vi "Auto Calibration.vi"(4 "Run Optimization Proc":bool, 5 "HasESI2":bool=TRUE, 6 "HasESI1":bool=TRUE, 7 "CalOption":enum32{"Positive", "Negative"}(radio)) -> (0 "error out":errorcluster)   [LabVIEW 2015]
uses:
  Type/_CalibrationStep.ctl
  Type/_GUI Method.ctl
  Type/_Lens Property.ctl
  Type/_Mass Range Property.ctl
  Type/_Mass Range Parameters.ctl
  Type/_RT Res Type.ctl
  Type/_Run Mode.ctl
  Type/_Instrument Model.ctl
  Controls/Auto-Detector Bias Info.ctl
  Controls/Auto-Detector Peak Info.ctl
  Type/_Log Command.ctl
  Type/_Data Operation.ctl
  Type/_RT Command.ctl
  Type/_CalibrationResult.ctl
  Type/_SaveOption.ctl
  Configuration/_Global Configuration.vi
  <vilib>/Utility/config.llb/Read Key (String).vi
  <vilib>/Utility/config.llb/Write Key (String).vi
  <vilib>/Utility/config.llb/NI_LVConfig.lvlib
panel:
  out "Q1 Data":string[][](array[string])
  out "Completed":bool=TRUE
  out "DV Optimization Run":string="Peak Width At (%): 50\nSearch Range (amu): +/- 2\nThreshold (counts): 1000\n"
  out "CalOption 2":enum32{"Positive", "Negative"}(ring)
  out "PeakWidth":cluster{"RefMass":dbl[], "PeakWidth":dbl[]}(graph) caption="EMS+Q1, Mass 59.06, EV30"
  out "MassShift":cluster{"RefMass":dbl[], "MassShift":dbl[]}(graph) caption="EMS+Q1, Mass 59.06, EV30"
  out "Resolution":string[][](table)=[["Quadrupole 1", "15"], ["Quadrupole 2", "3000"]]
  out "Iteration #":i32
  in  "Print":bool
  in  "Pause":bool
  out "Current Scan #":i32
  out "Calibration State":T1=enum."Get Cal Files"
  out "ScanMode":string="For Q1 Positive Mode"
  out "Detector":string[][](table)=[["Detector Deflector", "15"], ["Discriminator", "12"], ["Detector Voltage", "2350"], ["Detector Horn", "5500"]]
  out "Source":string[][](table)=[["Drying Gas", "40"], ["Nebulizer Gas 1", "0"], ["Heating Gas 1", "0"], ["Nebulizer Gas 2", "100"], ["Heating Gas 2", "0"], ["Source Exhaust", "0"], ["HSID Temperature", "200"], ["Source 1 Temp", "0"], ["Source 2 Temp", "0"], ["ElectroSpray V1", "3850"], ["ElectroSpray V2", "3850"], ["Curtain Cap", "1000"]]
  out "Instrument":string[][](table)=[["Multipole 1 RF", "350"], ["Entrance Voltage", "35"], ["Entrance Deflector", "0"], ["Multipole 1", "5"], ["Multipole Lens 1", "0"], ["Multipole 2", "0"], ["Multipole Lens 2", "0"], ["Prefilter", "-15"], ["Collision Cell Lens 1", "-10"], ["Collision Cell Lens 2", "-100"], ["Collision Energy", "-50"], ["Axial Field", "100"], ["Collision Cell Lens 3", "-120"], ["Collision Cell Lens 4", "-65"], ["Collision Pressure", "0"]]
  out "SearchParam":string="Peak Width At (%): 50\nSearch Range (amu): +/- 2\nThreshold (counts): 1000\n"
  out "SystemInfo":string="Instrument Model: IONICS 3Q 220\nInstrument Serial Number: A2103536\nManufacturer: PerkinElmer\nScan Mode: Q1, Positive\nResolution: Unit_Unit\nSource: ESI2\nMethod: +Q1 PPG"
  out "DateLabel":string="Date Performed: 10/08/2013 09:12:58\nLast Performed: 09/12/2013 14:12:55"
  out "Pages":enum32{"Page 1", "Page 2", "Page 3", "Page 4"}(tab)
  out "MR 8":cluster{dbl[], dbl[]}(graph)
  out "MR 7":cluster{dbl[], dbl[]}(graph) caption="Q2 Pos, Mass 1545.13, EV70"
  out "MR 6":cluster{dbl[], dbl[]}(graph) caption="Q2 Pos, Mass 906.67, EV55"
  out "MR 5":cluster{dbl[], dbl[]}(graph) caption="Q2 Pos, Mass 616.46, EV55"
  out "MR 4":cluster{dbl[], dbl[]}(graph) caption="Q2 Pos, Mass 384.30, EV0"
  out "MR 3":cluster{dbl[], dbl[]}(graph) caption="Q2 Pos, Mass 175.13, EV55"
  out "MR 2":cluster{dbl[], dbl[]}(graph) caption="Q2 Pos, Mass 117.09, EV55"
  out "Current Results":string[][](table) caption="02/16/2017 10:53:40"
  out "MR 1":cluster{dbl[], dbl[]}(graph) caption="Q2 Pos, Mass 59.05, EV55"
  out "Previous Auto Calibration Results":string[][](table) caption="02/13/2017 14:08:53"
  out "ParmeterFolder":path
  out "ResolutionFile":path
  out "ReportFolder":path
  out "Q2ReportPage":path
  out "Q1ReportPage":path
  out "Init":bool
  out "Model Name":T2=enum."IONICS 3Q 210"
  out "UsingESI1":bool=TRUE
  out "Quit":bool
  out "oldTablePath":path
  out "Q1 Method":path=path "C:/Users/Min/Projects/SVN/Sniffer900/Release/Ionics Service Tool/Q1PositiveMethod.d2m"
  out "Q2 Method":path=path "C:/Users/Min/Projects/SVN/Sniffer900/Release/Ionics Service Tool/Q1NegativeMethod.d2m"
  in  "Page":bool=TRUE
  in  "GotoPg2":bool
  in  "GotoPg1":bool
  out "PeakSearchParameters":dbl[](array[numeric])
  out "MassReference":cluster{"Mass":dbl, "Use":bool}[](array[cluster])
  out "Method":T3={"Lenses"=[], "Mass Ranges"=[], "Acquire"=FALSE, "MCA"=FALSE, "Q1DC EN"=FALSE, "Q1 POL"=FALSE, "Q3 POL"=FALSE, "Q1 RF  EN"=FALSE, "Averaging"=FALSE, "Log Scale"=FALSE, "CPS"=FALSE, "Unit"=FALSE, "Data Path"=path "", "Run Mode"=enum."MRM (Q1/Q2)", "Fixed Mass (amu)"=1.0, "Q3DC EN"=FALSE, "Q3 RF  EN"=FALSE, "Negative"=FALSE} {"Mass Ranges"."Res" items=["High/High", "Medium/Medium", "Low/Low", "High/Medium", "High/Low", "Medium/High", "Medium/Low", "Low/High", "Low/Medium"]}
  # "Auto CAL/RES Results Report"
  # "System Information"
  # "Search Parameters"
  # "Number of Scans (Sum): 10"
  # "Page 3"
  # "Page 4"
  # "MinimumMassPeakWidth"
  # "ThresholdForMassSpectrum"
  # "SearchRange"
  # "NumberOfSmooth"
  # "NumberOfPointsToSmooth"
  # "WidthAtOfMaximum"
  # "PeakFindingNoiseLevel"
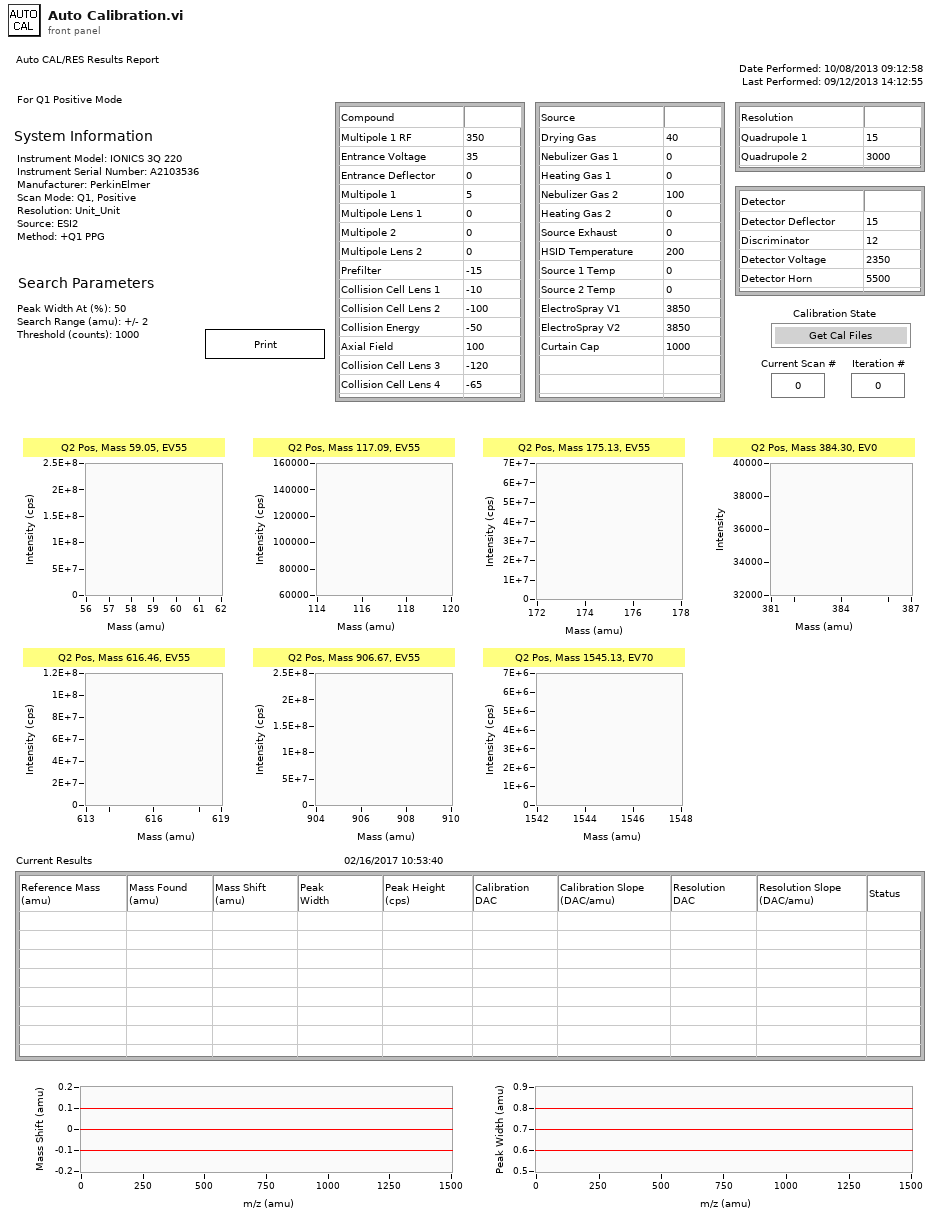
[diagram p1: front panel]
types:
  T1 = typedef "_CalibrationStep.ctl" = enum16{"Export Optimization", "Get Cal Files", "Read Q1 Method", "Acquire Q1 Data", "Process Q1 Data", "Generate Report", "Prepare For Q2 Cal", "Read Q2 Method", "Acquire Q2 Data", "Process Q2 Data", "Done", "Pause"}
  T2 = typedef "_Instrument Model.ctl" = enum16{"QSight 110", "QSight 120", "QSight 210", "QSight 220", "IONICS 3Q 110", "IONICS 3Q 120", "IONICS 3Q 210", "IONICS 3Q 220", "IONICS 3Q 310", "IONICS 3Q 320", "Simulation (Single Source)", "Simulation (Dual Source)"}
  T3 = typedef "_GUI Method.ctl" = cluster{"Lenses":T4[], "Mass Ranges":T5[], "Acquire":bool, "MCA":bool, "Q1DC EN":bool, "Q1 POL":bool, "Q3 POL":bool, "Q1 RF  EN":bool, "Averaging":bool, "Log Scale":bool, "CPS":bool, "Unit":bool, "Data Path":path, "Run Mode":T8, "Fixed Mass (amu)":dbl, "Q3DC EN":bool, "Q3 RF  EN":bool, "Negative":bool}
  T4 = typedef "_Lens Property.ctl" = cluster{"Scan Type":u8, "Scans":i32, "Time 1":dbl, "Time 2":dbl, "Value 1":dbl, "Value 2":dbl, "Step Size":dbl}
  T5 = typedef "_Mass Range Property.ctl" = cluster{"Start":dbl, "Stop":dbl, "Step Size":dbl, "Steps":i32, "Dwell":dbl, "Parameters":T6[], "Res":T7}
  T6 = typedef "_Mass Range Parameters.ctl" = cluster{"Name":string, "Ch#":u8, "StartV":dbl, "StopV":dbl, "StepV":dbl, "Index":u8}
  T7 = typedef "_RT Res Type.ctl" = u16
  T8 = typedef "_Run Mode.ctl" = enum16{"MRM (Q1/Q2)", "Q1 Scan", "Q1 SRM", "Q2 Scan", "Q2 SRM", "Product Scan", "Precursor Scan", "Neutral Loss", "Neutral Gain"}
  T9 = typedef "Auto-Detector Peak Info.ctl" = cluster{"Run Bias":u32, "Peak Height":dbl, "% Increase":dbl, "Peak Found":bool}
  T10 = typedef "Auto-Detector Bias Info.ctl" = cluster{"Run Optimization Proc":bool, "Optimization Run Bias":u32, "Run Bias Info":T9[]}
  T11 = typedef "_CalibrationResult.ctl" = cluster{"RefMass":dbl, "MassFound":dbl, "MassShift":dbl, "PeakWidth":dbl, "CalDAC":dbl, "CalSlope":dbl, "ResDAC":dbl, "ResSlope":dbl, "Status":enum16{"Found", "Missing", "Not Used"}, "CalOK":bool, "ResOK":bool, "PeakHeight":dbl}
  T12 = typedef "_Log Command.ctl" = enum16{"No Command", "Open", "Read", "Write", "Close", "Check Size"}
  T13 = typedef "_RT Command.ctl" = enum16{"xml Start Run", "xml Start Actual Run", "xml Stop Run", "xml Runtime Update", "xml Get Status", "xml Get Table", "xml Set Table", "xml Get Configuration", "xml System Status", "xml Set LC Input Logic", "xml Get Data", "xml Get Info", "Start", "StartActualRun", "Stop", "Runtime Update", "Get Data", "Get Info", "Get Status", "Get Param", "Get Config", "Get Table", "Read ADC", "Set Oscillator", "Update Config", "Update Table", "Set All Pol", "Set Pol and DC", "Set Max Mass", "Toggle RP", "Toggle EL", "Set PIC", "Initialize Turbo", "Send Turbo Comm", "Close Turbo", "P1", "P2", "P3", "Send Serial", "Set LC Out", "Get LC In", "Read VAC", "Test Table", "Toggle Power", "Get Startup", "Set Startup", "Get ADC Table", "Set ADC Table", "Get Brief Status", "Get Detail Status", "Auxiliary Update", "Set CC Logics", "Set CC Input Logics", "Ignore Error", "invalid"}
  T14 = typedef "_SaveOption.ctl" = enum16{"Use Dialog", "Temporary File", "My Tables", "Full Path"}
  T15 = typedef "_Data Operation.ctl" = enum8{"Initialize", "Get Data", "Set Data", "Close"}
  T16 = typedef "NI_LVConfig.lvlib/Config Data RefNum.ctl" = refnum<k1>
  T17 = typedef "imagedata.ctl" = cluster{"image type":i32, "image depth":i32, "image":u8[], "mask":u8[], "colors":u32[], "Rectangle":cluster{"left":i16, "top":i16, "right":i16, "bottom":i16}}
  T18 = enum16{"Left Button", "Center Button", "Right Button", "Window Close"}
  T19 = typedef "_Current Data.ctl" = cluster{"Scan#":i32, "Run Time (mS)":i32, "TIC X":dbl[], "TIC Y":dbl[][], "MassRange":cluster{"X Title":string, "X":dbl[], "Y":i32[]}[], "Fixed Mass (amu)":dbl, "Method":T20}
  T20 = typedef "_XML Expt.ctl" = cluster{"StartT(mS)":i32, "#Cycles":i32, "PauseT(uS)":i32, "ScanType":i32, "Polarity":u8, "FixedMass":dbl, "DelayT(mS)":i32, "Active Ch":T21[], "Mass Range":T5[]}
  T21 = typedef "_XML Lens.ctl" = cluster{"Value":dbl, "ChID":u8}
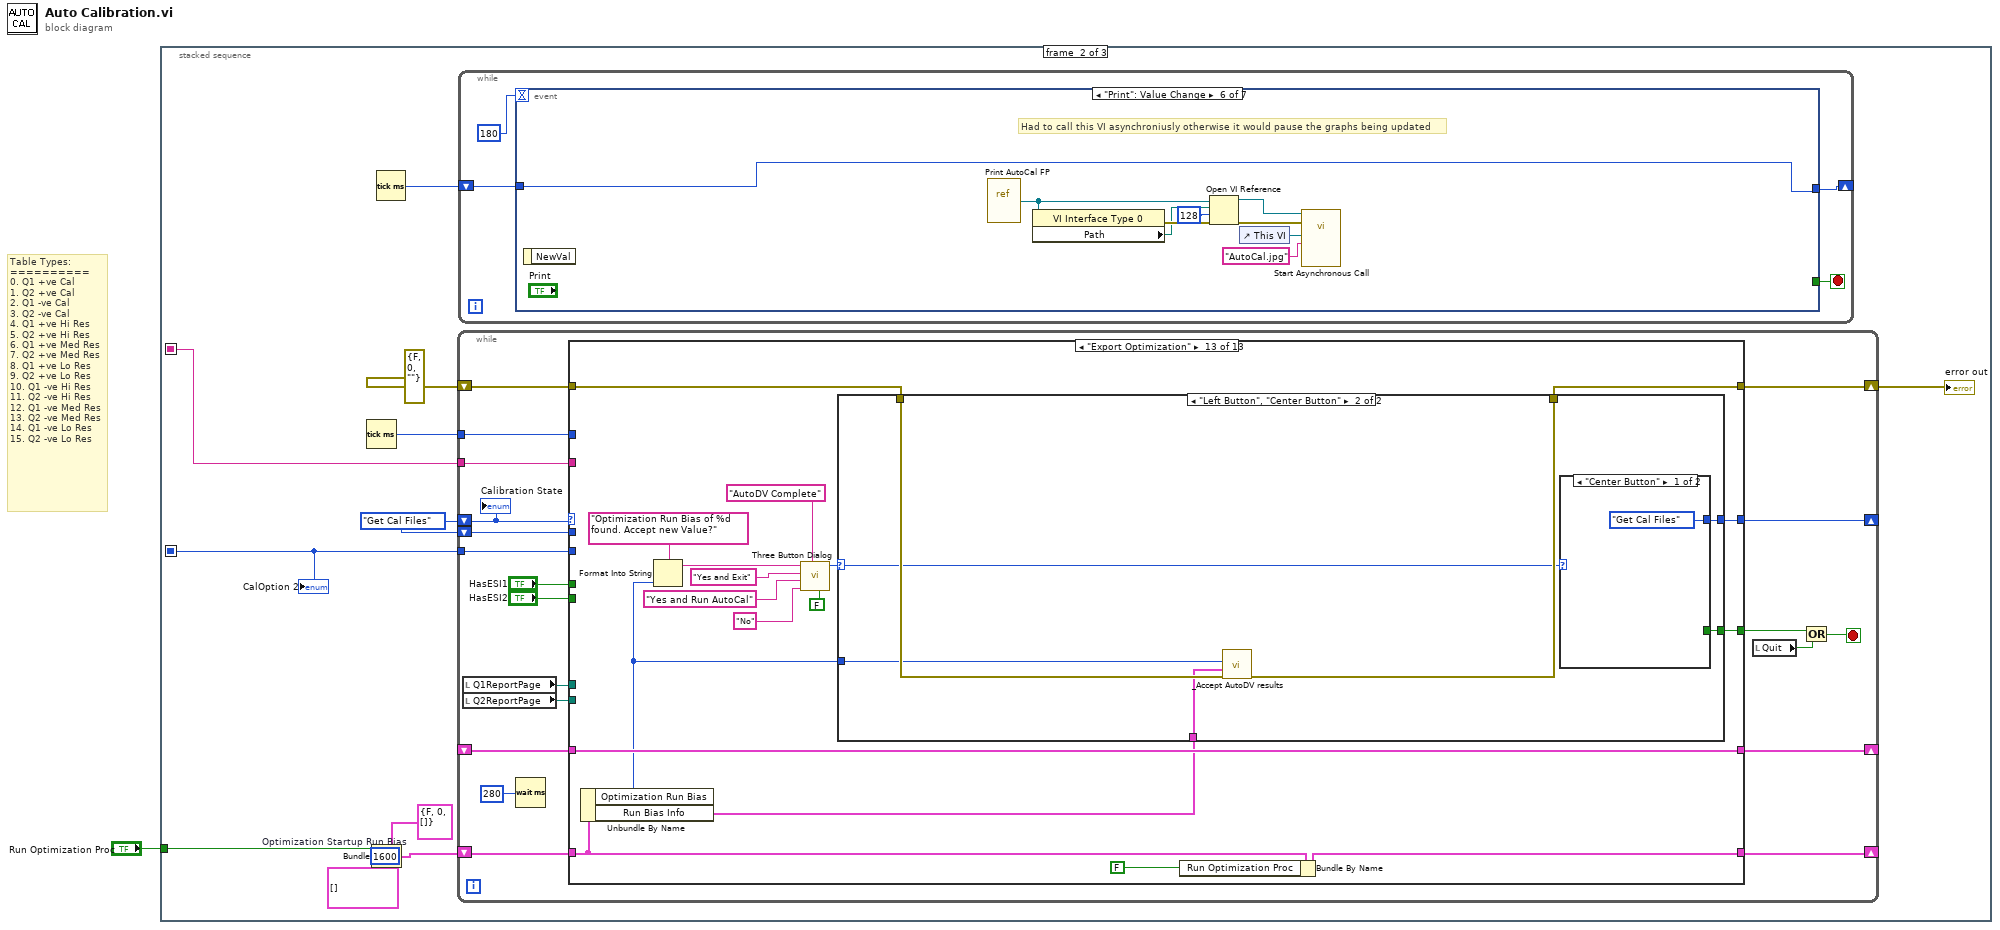
[diagram p0: block diagram]
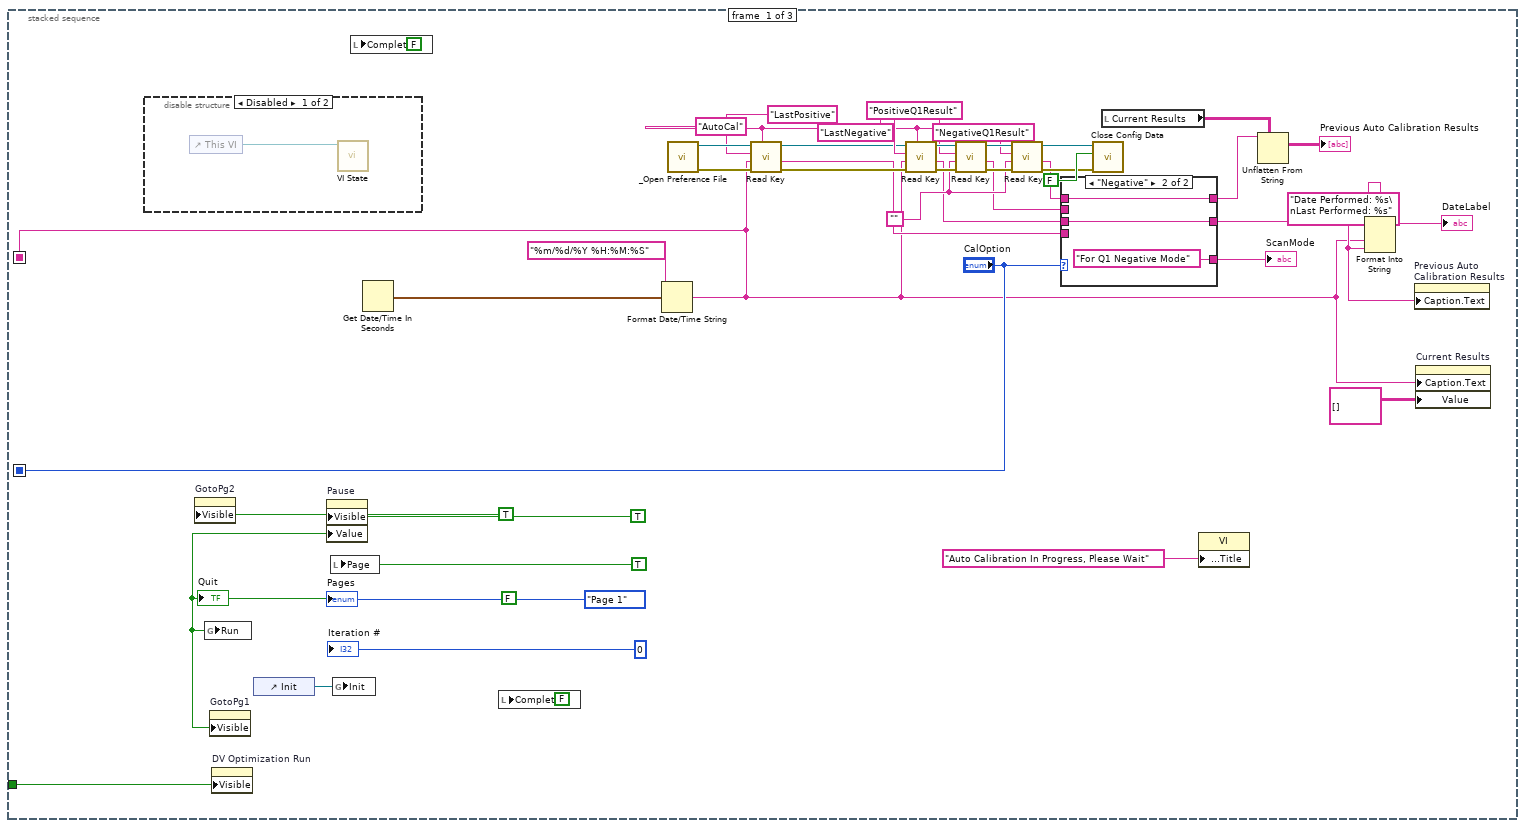
[diagram p2: hidden frame]
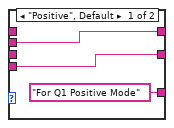
[diagram p4: hidden frame]
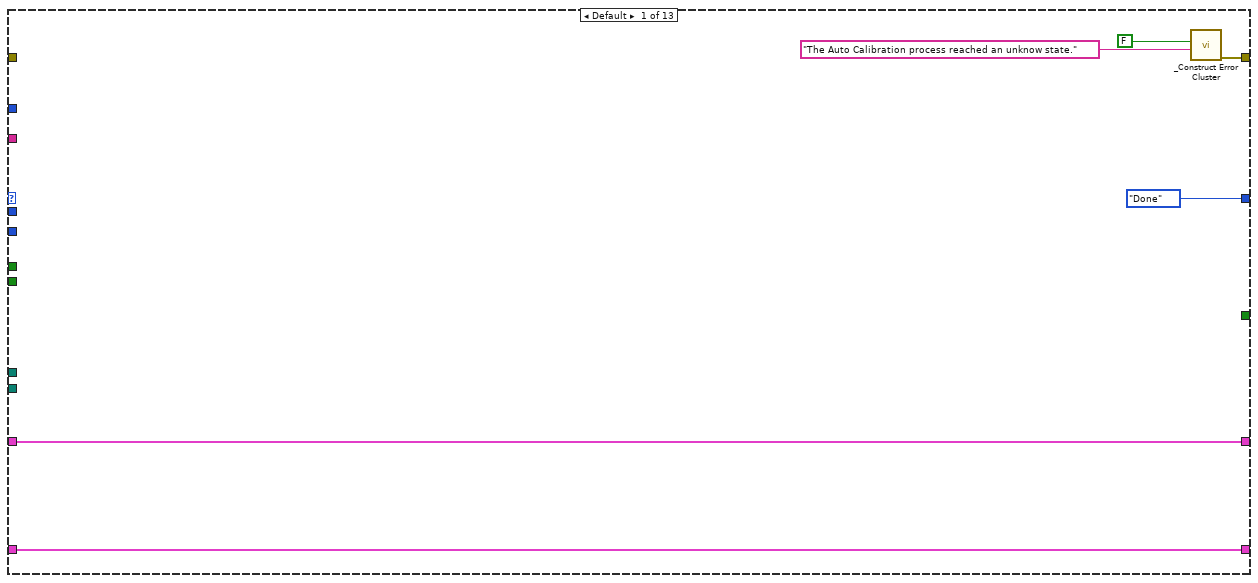
[diagram p5: hidden frame]
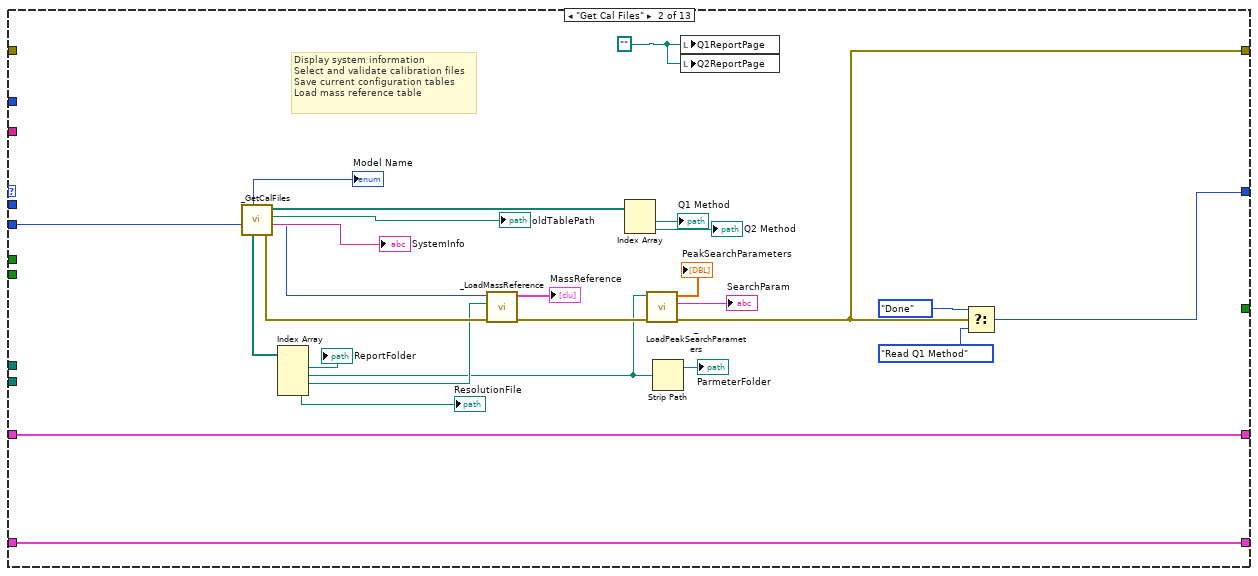
[diagram p6: hidden frame]
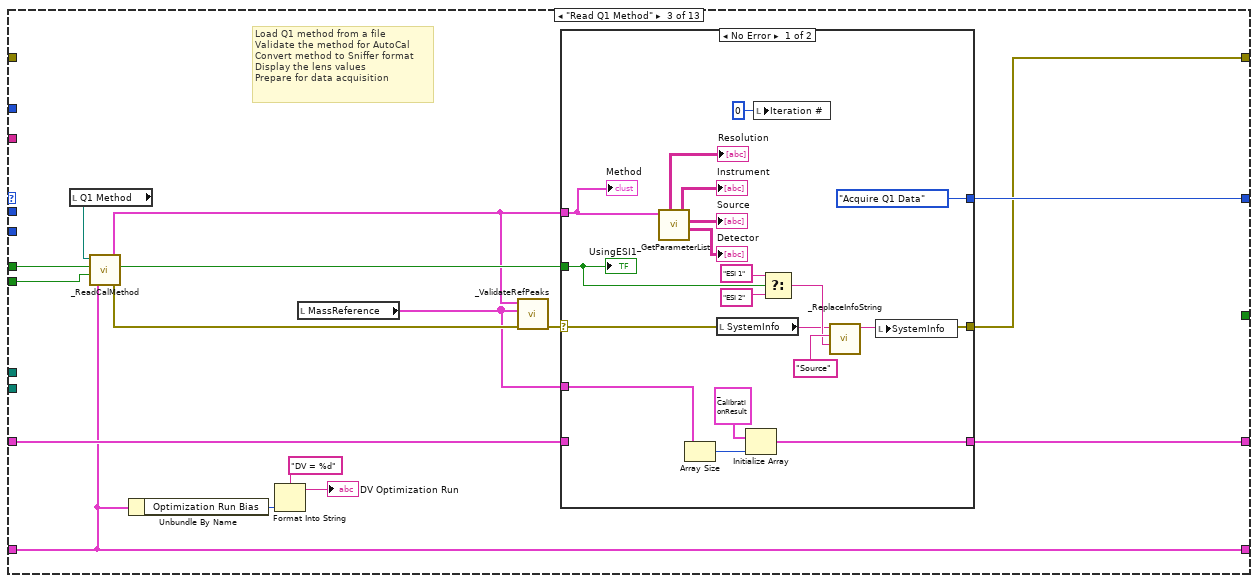
[diagram p7: hidden frame]
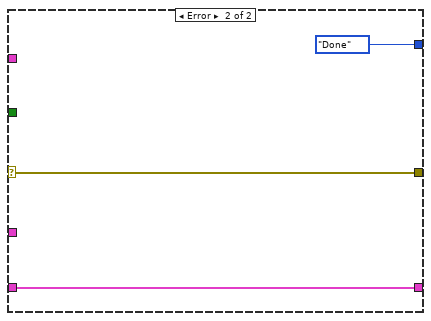
[diagram p8: hidden frame]
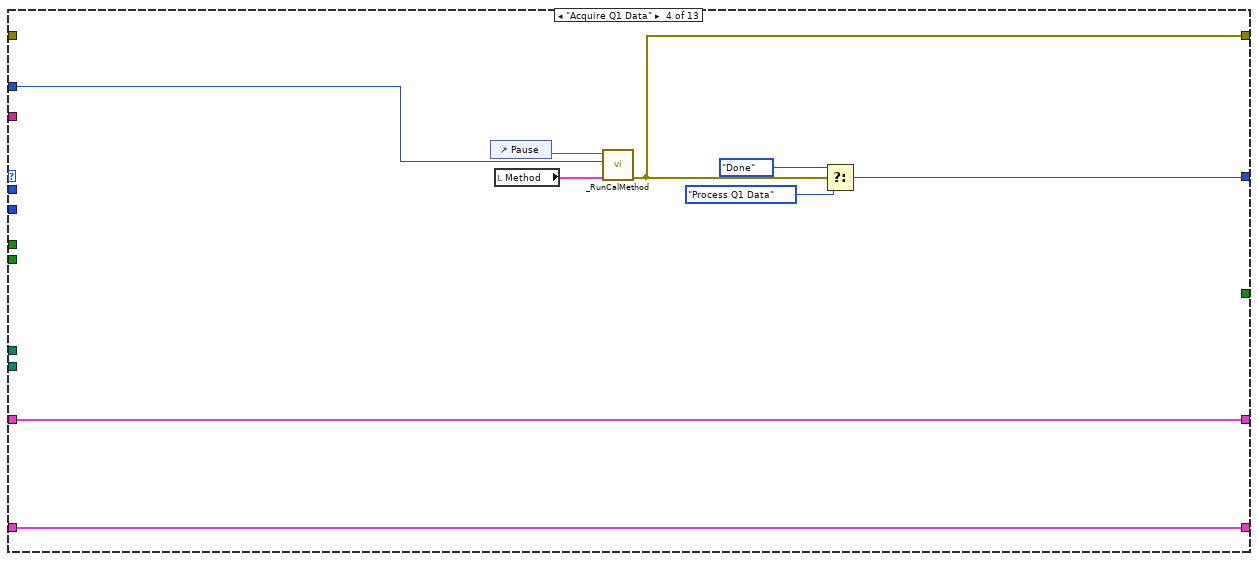
[diagram p9: hidden frame]
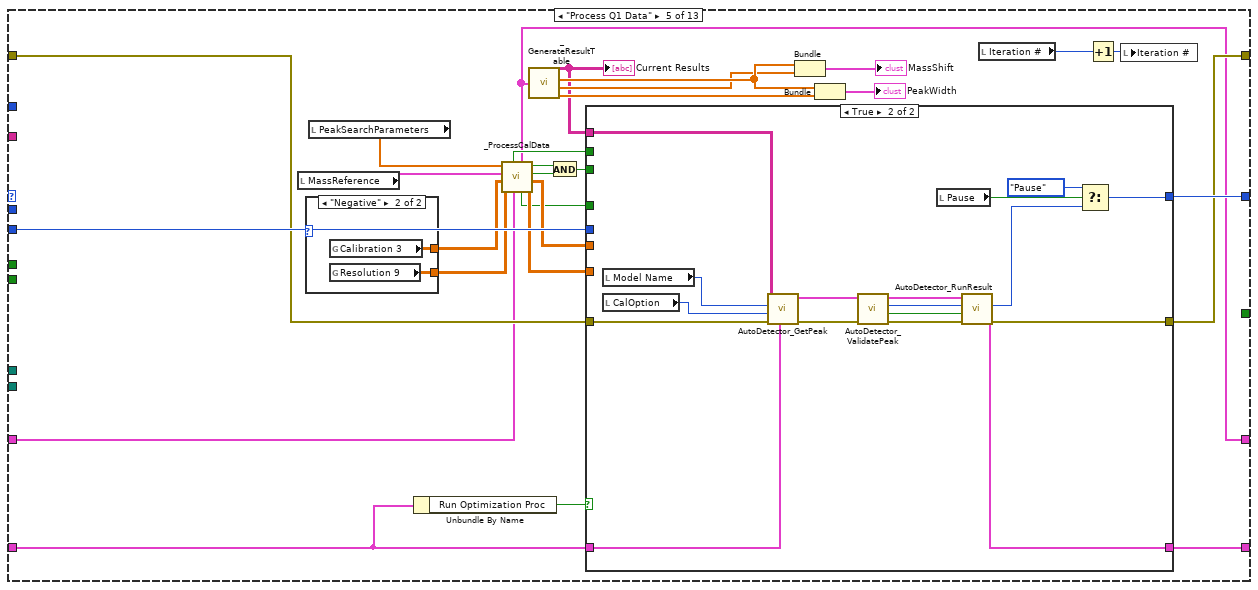
[diagram p10: hidden frame]
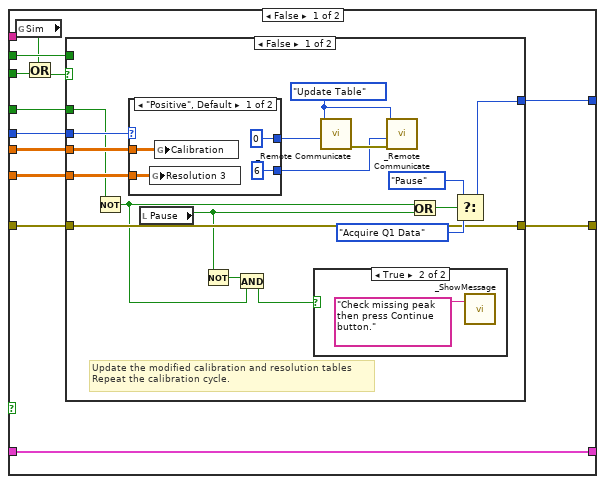
[diagram p11: hidden frame]
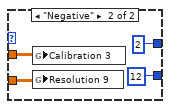
[diagram p13: hidden frame]
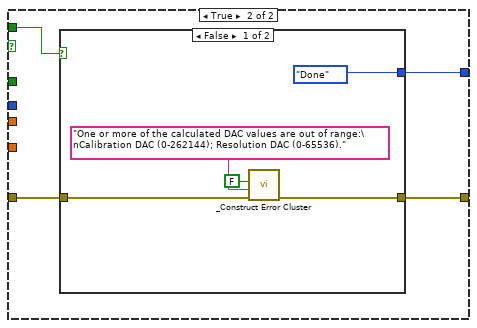
[diagram p14: hidden frame]
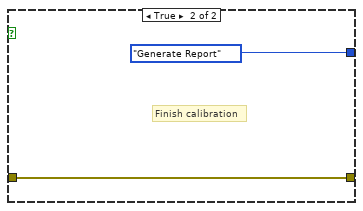
[diagram p15: hidden frame]
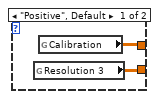
[diagram p16: hidden frame]
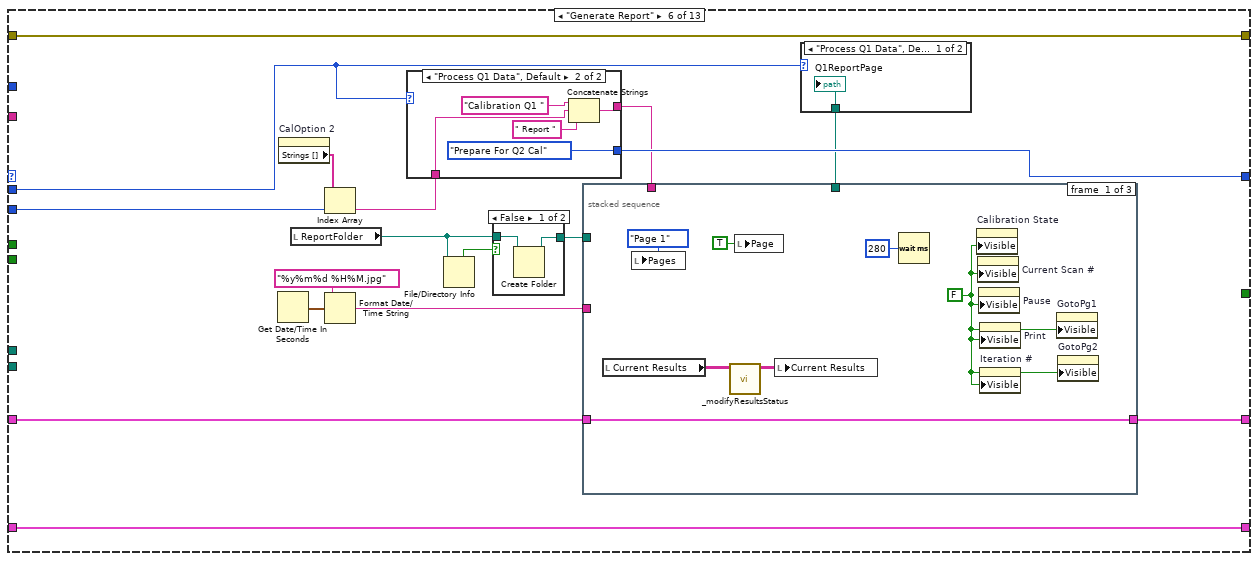
[diagram p17: hidden frame]
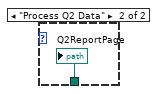
[diagram p18: hidden frame]
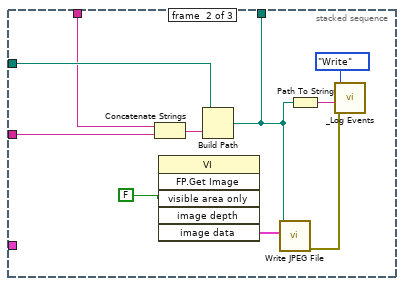
[diagram p20: hidden frame]
diagram:
  # "Table Types:\n==========\n0. Q1 +ve Cal\n1. Q2 +ve Cal\n2. Q1 -ve Cal\n3. Q2 -ve Cal\n4. Q1 +ve Hi Res\n5. Q2 +ve Hi Res\n6. Q1 +ve Med Res\n7. Q2 +ve Med Res\n8. Q1 +ve Lo Res\n9. Q2 +ve Lo Res\n10. Q1 -ve Hi Res\n11. Q2 -ve Hi Res\n12. Q1 -ve Med Res\n13. Q2 -ve Med Res\n14. Q1 -ve Lo Res\n15. Q2 -ve Lo Res"
  n1 = stacked-sequence {
    seq-local: ["CalOption" _ _] -> [_ w64 w667]
    seq-local: [w13 _ _] -> [_ w61 _]
    tunnel: "Run Optimization Proc" -> [w4 w54 _]
    frame #0 {
      w26 = ""
      w30 = "AutoCal" ("section")
      w6 = FALSE ("Quit")
      n2 = disable-structure shown="Disabled" {
        frame Disabled {
          n3 = control-ref of="This VI"() -> (w46:refnum<vi>)
          n4 = call "VI State.vi"("VI in"=w46) -> ()  [unwired: 10 in, 1 out]
        }
        frame Enabled {
        }
      }
      n5 = property on="GotoPg2" class="Bool"("Visible"=TRUE) -> ()  [unwired: 2 in, 2 out]
      n6 = global write "_Global Configuration.vi" "Run"(w6) -> ()
      n7 = property on="GotoPg1" class="Bool"("Visible"=w6) -> ()  [unwired: 2 in, 2 out]
      n8 = property on="DV Optimization Run" class="Str"("Visible"=w4) -> ()  [unwired: 2 in, 2 out]
      n9 = control-ref of="Init"() -> (w12:refnum<vi>)
      n10 = property on="Pause" class="Bool (strict)"("Visible"=TRUE, "Value"=w6) -> ()  [unwired: 2 in, 2 out]
      n11 = local write "Page"(TRUE ("Page")) -> ()
      n12 = global write "_Global Configuration.vi" "Init"(w12) -> ()
      n13 = local write "Completed"(FALSE ("Accepted")) -> ()
      n14 = Get Date/Time In Seconds() -> (seconds since 1Jan1904=w37:timestamp)
      n15 = local write "Completed"(FALSE ("Accepted")) -> ()
      n16 = Format Date/Time String(time format string (%c)="%m/%d/%Y %H:%M:%S", seconds (now)=w37) -> (date/time string=w13:string)  [unwired: 1 in]
      n17 = call "_Open Preference File.vi"() -> ("error"=w40:errorcluster, "refnum"=w44:T16)  [unwired: 3 in, 3 out]
      n18 = call-poly <vilib>:"Read Key.vi"("section"=w30, "error in (no error)"=w40, "default value"=w13, "key"="LastPositive" ("section"), "refnum"=w44) -> ("error out"=w39:errorcluster, "value"=w22:string, "refnum out"=w41:T16)  [unwired: 3 in, 1 out]
      n19 = call-poly <vilib>:"Read Key.vi"("section"=w30, "error in (no error)"=w39, "default value"=w13, "key"="LastNegative" ("section"), "refnum"=w41) -> ("error out"=w35:errorcluster, "value"=w23:string, "refnum out"=w34:T16)  [unwired: 3 in, 1 out]
      n20 = call-poly <vilib>:"Read Key.vi"("section"=w30, "error in (no error)"=w35, "default value"=w26, "key"="PositiveQ1Result" ("section"), "refnum"=w34) -> ("error out"=w32:errorcluster, "value"=w24:string, "refnum out"=w31:T16)  [unwired: 3 in, 1 out]
      n21 = call-poly <vilib>:"Read Key.vi"("section"=w30, "error in (no error)"=w32, "default value"=w26, "key"="NegativeQ1Result" ("section"), "refnum"=w31) -> ("error out"=w27:errorcluster, "value"=w25:string, "refnum out"=w28:T16)  [unwired: 3 in, 1 out]
      n22 = case shown="\"Negative\"" "CalOption" {
        tunnel: w25 -> [_ w51]
        tunnel: w24 -> [w48 _]
        tunnel: w23 -> [_ w50]
        tunnel: w22 -> [w47 _]
        tunnel: ["For Q1 Positive Mode" ("ScanMode") "For Q1 Negative Mode" ("ScanMode")] -> w21
        tunnel: [w48 w51] -> w19
        tunnel: [w47 w50] -> w15
        frame "Positive", Default {
        }
        frame "Negative" {
        }
      }
      "ScanMode" <- w21
      n23 = call <vilib>:"Close Config Data.vi"("error in (no error)"=w27, "write file if changed (T)"=FALSE, "refnum"=w28) -> ()  [unwired: 9 out]
      n24 = local read "Current Results"() -> (w20:string[][])
      n25 = property class="VI"("Front Panel Window:Title"="Auto Calibration In Progress, Please Wait") -> ()  [unwired: 2 in, 2 out]
      n26 = Unflatten From String(type=w20, binary string=w19) -> (value=→"Previous Auto Calibration Results":string[][])  [unwired: 3 in, 2 out]
      n27 = Format Into String(format string="Date Performed: %s\nLast Performed: %s", w13, w15) -> (resulting string=→"DateLabel":string)  [unwired: 2 in, 1 out]
      n28 = property on="Previous Auto Calibration Results" class="Tbl (strict)"("Caption.Text"=w15) -> ()  [unwired: 2 in, 2 out]
      n29 = property on="Current Results" class="Tbl (strict)"("Caption.Text"=w13, "Value"=string[][] [] ("Current Results")) -> ()  [unwired: 2 in, 2 out]
      "Quit" <- w6
      "Pages" <- enum32{"Page 1", "Page 2", "Page 3", "Page 4"}."Page 1" ("Pages")
      "Iteration #" <- 0 ("Iteration #")
    }
    frame #1 {
      w58 = u32 1600  # Optimization Startup Run Bias
      w62 = _CalibrationStep."Get Cal Files" ("f")
      n30 = Tick Count (ms)() -> (millisecond timer value=w55:u32)
      n31 = Bundle(cluster=T10 {"Run Optimization Proc"=FALSE, "Optimization Run Bias"=0, "Run Bias Info"=[]}, "Run Optimization Proc"=w54, "Optimization Run Bias"=w58, "Run Bias Info"=T9[] []) -> (w60:T10)
      n32 = Tick Count (ms)() -> (millisecond timer value=w53:u32)
      n33 = while {
        shift-right: [w84] -> _
        shift-left: w62 -> [w82]
        tunnel: w64 -> [w78]
        shift-right: [w76] -> w56
        shift-left: errorcluster {"status"=FALSE, "code"=0, "source"=""} ("error out 2") -> [w77]
        shift-left: w62 -> [w73]
        tunnel: w61 -> [w72]
        shift-right: [w71] -> _
        shift-left: _ -> [w70]
        shift-right: [w66] -> _
        shift-left: w60 -> [w67]
        tunnel: w55 -> [w65]
        stop <- w79 stop-if-true
        n34 = local read "Q1ReportPage"() -> (w69:path)
        n35 = local read "Q2ReportPage"() -> (w68:path)
        n36 = Wait (ms)(milliseconds to wait=u32 280) -> ()  [unwired: 1 out]
        n37 = case shown="\"Export Optimization\"" w82 {
          selector: w82 -> [_ _ _ _ _ _ _ _ _ _ w461 _ _]
          tunnel: [_CalibrationStep."Done" ("f") w112 w131 w160 w174 w276 _CalibrationStep."Read Q2 Method" ("f") w354 w383 w397 w461 w524 w550] -> w84
          tunnel: [_ _ _ _ _ _ _ _ _ _ w463 w523 w538] -> w81
          tunnel: w78 -> [_ w106 _ _ w188 w265 w332 _ _ w411 w465 _ _]
          tunnel: w77 -> [_ _ _ _ w171 w277 w333 _ _ w394 w462 w526 w549]
          tunnel: [w88 w103 w120 w161 w172 w277 w333 w342 w384 w395 w462 w526 w548] -> w76
          tunnel: "HasESI1" -> [_ _ w129 _ _ _ _ w352 _ _ _ _ _]
          tunnel: "HasESI2" -> [_ _ w128 _ _ _ _ w351 _ _ _ _ _]
          tunnel: w73 -> [_ _ _ _ _ w269 _ _ _ _ w460 w525 _]
          tunnel: w72 -> [_ _ _ _ _ _ _ _ _ _ w455 _ _]
          tunnel: [w86 w100 w123 w158 w168 w261 w314 w345 w381 w390 w459 w522 w555] -> w71
          tunnel: w70 -> [w86 w100 w124 w158 w167 w262 w314 w347 w381 w391 w459 w522 w555]
          tunnel: w69 -> [_ _ _ _ _ _ _ _ _ _ w457 _ _]
          tunnel: w68 -> [_ _ _ _ _ _ _ _ _ _ w458 _ _]
          tunnel: w67 -> [w85 w92 w119 w157 w163 w263 w313 w344 w380 w389 w456 w521 w554]
          tunnel: [w85 w92 w119 w157 w164 w263 w313 w344 w380 w389 w456 w521 w552] -> w66
          tunnel: w65 -> [_ _ _ w154 _ _ _ _ w377 _ _ _ _]
          frame Default {
            n38 = call "_Construct Error Cluster.vi"("reason"="The Auto Calibration process reached an unknow state.", "CallingChain? (T)"=FALSE) -> ("error out"=w88:errorcluster)  [unwired: 5 in]
          }
          frame "Get Cal Files" {
            w99 = path ""
            # "Display system information\nSelect and validate calibration files\nSave current configuration tables\nLoad mass reference table"
            n39 = call "_GetCalFiles.vi"("CalOption"=w106) -> ("error out"=w107:errorcluster, "SystemInfo"=→"SystemInfo":string, "oldTablePath"=→"oldTablePath":path, "calFiles"=w111:path[], "OtherDirectories"=w98:path[], "Model Name"=→"Model Name":T2)  [unwired: 3 in]
            n40 = Index Array(array=w98) -> (element #1=→"ReportFolder":path, element #2=w94:path, element #3=w97:path, element #4=→"ResolutionFile":path)  [unwired: 4 in]
            n41 = call "_LoadMassReference.vi"("error in (no error)"=w107, "Path"=w97, "Polarity"=w106) -> ("error out"=w104:errorcluster, "MassReference"=→"MassReference":cluster{"Mass":dbl, "Use":bool}[])  [unwired: 3 in]
            n42 = Index Array(array=w111) -> (element #1=→"Q1 Method":path, element #2=→"Q2 Method":path)  [unwired: 2 in]
            n43 = call "_LoadPeakSearchParameters.vi"("error in (no error)"=w104, "Path"=w94) -> ("error out"=w103:errorcluster, "SearchParameters"=→"SearchParam":string, "PeakSearchParameters"=→"PeakSearchParameters":dbl[])  [unwired: 3 in]
            n44 = Strip Path(path=w94) -> (stripped path=→"ParmeterFolder":path)  [unwired: 1 out]
            n45 = local write "Q1ReportPage"(w99) -> ()
            n46 = local write "Q2ReportPage"(w99) -> ()
            n47 = Select(t=_CalibrationStep."Done" ("f"), s=w103, f=_CalibrationStep."Read Q1 Method") -> (s? t:f=w112:T1)
          }
          frame "Read Q1 Method" {
            # "Load Q1 method from a file\nValidate the method for AutoCal\nConvert method to Sniffer format\nDisplay the lens values\nPrepare for data acquisition"
            n48 = local read "Q1 Method"() -> (w121:path)
            n49 = call "_ReadCalMethod.vi"("Auto-Detect Bias info"=w119, "HasESI2"=w128, "HasESI1"=w129, "Method Path"=w121) -> ("error out"=w127:errorcluster, "UseESI1"=w130:bool, "GUI Method"=w126:T3)  [unwired: 1 in]
            n50 = Unbundle By Name(w119) -> ("Optimization Run Bias"=w117:u32)
            n51 = Format Into String(format string="DV = %d", w117) -> (resulting string=→"DV Optimization Run":string)  [unwired: 2 in, 1 out]
            n52 = local read "MassReference"() -> (w122:cluster{"Mass":dbl, "Use":bool}[])
            n53 = call "_ValidateRefPeaks.vi"("error in (no error)"=w127, "MassReference"=w122, "Method"=w126) -> ("error out"=w125:errorcluster)  [unwired: 4 in]
            n54 = case shown="No Error" w125 {
              selector: w125 -> [w132 w151]
              tunnel: [_CalibrationStep."Acquire Q1 Data" ("f") _CalibrationStep."Done" ("f")] -> w131
              tunnel: w126 -> [w149 _]
              tunnel: w130 -> [w144 _]
              tunnel: w124 -> [_ w152]
              tunnel: [w133 w152] -> w123
              tunnel: w122 -> [w136 _]
              tunnel: [w132 w151] -> w120
              frame No Error {
                n55 = call "_GetParameterList.vi"("GUI Method"=w149) -> ("Detector"=→"Detector":string[][], "Source"=→"Source":string[][], "Instrument"=→"Instrument":string[][], "Resolution"=→"Resolution":string[][])  [unwired: 3 in, 1 out]
                n56 = Array Size(array=w136) -> (size(s)=w135:i32)
                n57 = local read "SystemInfo"() -> (w139:string)
                n58 = Initialize Array(T11 {"RefMass"=0.0, "MassFound"=0.0, "MassShift"=0.0, "PeakWidth"=0.0, "CalDAC"=0.0, "CalSlope"=0.0, "ResDAC"=0.0, "ResSlope"=0.0, "Status"=enum."Found", "CalOK"=FALSE, "ResOK"=FALSE, "PeakHeight"=0.0} ("CalResult"), w135) -> (w133:T11[])
                n59 = local write "Iteration #"(0 ("Iteration #")) -> ()
                n60 = Select(t="ESI 1", s=w144, f="ESI 2") -> (s? t:f=w140:string)
                n61 = call "_ReplaceInfoString.vi"("Value"=w140, "Key"="Source", "SystemInfo"=w139) -> ("SystemInfoOut"=w145:string)  [unwired: 4 in]
                n62 = local write "SystemInfo"(w145) -> ()
                "Method" <- w149
                "UsingESI1" <- w144
              }
              frame Error {
              }
            }
          }
          frame "Acquire Q1 Data" {
            n63 = control-ref of="Pause"() -> (w159:refnum<vi>)
            n64 = local read "Method"() -> (w162:T3)
            n65 = call "_RunCalMethod.vi"("Method"=w162, "millisecond timer value"=w154, "Pause"=w159) -> ("error out"=w161:errorcluster)  [unwired: 4 in]
            n66 = Select(t=_CalibrationStep."Done", s=w161, f=_CalibrationStep."Process Q1 Data") -> (s? t:f=w160:T1)
          }
          frame "Process Q1 Data" {
            n67 = local read "MassReference"() -> (w189:cluster{"Mass":dbl, "Use":bool}[])
            n68 = case shown="\"Negative\"" w188 {
              tunnel: [w258 w260] -> w187
              tunnel: [w257 w259] -> w186
              frame "Positive", Default {
                n69 = global read "_Global Configuration.vi" "Resolution 3"() -> (w257:dbl[][])
                n70 = global read "_Global Configuration.vi" "Calibration"() -> (w258:dbl[][])
              }
              frame "Negative" {
                n71 = global read "_Global Configuration.vi" "Calibration 3"() -> (w260:dbl[][])
                n72 = global read "_Global Configuration.vi" "Resolution 9"() -> (w259:dbl[][])
              }
            }
            n73 = local read "PeakSearchParameters"() -> (w190:dbl[])
            n74 = Unbundle By Name(w163) -> ("Run Optimization Proc"=w165:bool)
            n75 = call "_ProcessCalData.vi"("CalResultIn"=w167, "Resolution"=w186, "Calibration"=w187, "MassReference"=w189, "PeakSearchParameters"=w190) -> ("ResolutionOut"=w184:dbl[][], "CalibrationOut"=w185:dbl[][], "ResOK"=w182:bool, "CalOK"=w183:bool, "AllFound"=w175:bool, "CalResultOut"=w168:T11[], "AllValid"=w173:bool)
            n76 = call "_GenerateResultTable.vi"("CalResults"=w168) -> ("ResultTable"=w166:string[][], "RefMass"=w178:dbl[], "MassShift"=w177:dbl[], "PeakWidth"=w180:dbl[])
            "Current Results" <- w166
            n77 = And(x=w183, y=w182) -> (x .and. y?=w181:bool)
            n78 = case shown="True" w165 {
              tunnel: w188 -> [w202 _]
              tunnel: w185 -> [w201 _]
              tunnel: w184 -> [w200 _]
              tunnel: w181 -> [w199 _]
              tunnel: w175 -> [w198 _]
              tunnel: [w197 w242] -> w174
              tunnel: w173 -> [w196 _]
              tunnel: [w195 w249] -> w172
              tunnel: w171 -> [w194 w256]
              tunnel: w166 -> [_ w255]
              tunnel: [w193 w245] -> w164
              tunnel: w163 -> [w193 w246]
              frame False {
                n79 = global read "_Global Configuration.vi" "Sim"() -> (w191:bool)
                n80 = Or(x=w191, y=w199) -> (x .or. y?=w192:bool)
                n81 = case shown="False" w192 {
                  tunnel: w202 -> [w219 _]
                  tunnel: w201 -> [w218 _]
                  tunnel: w200 -> [w217 _]
                  tunnel: [w210 w232] -> w197
                  tunnel: w198 -> [w209 _]
                  tunnel: w196 -> [_ w231]
                  tunnel: [w207 w230] -> w195
                  tunnel: w194 -> [w207 w229]
                  frame False {
                    w215 = _RT_Command."Update Table" ("Command")
                    # "Update the modified calibration and resolution tables\nRepeat the calibration cycle."
                    n82 = Not(x=w209) -> (.not. x?=w204:bool)
                    n83 = case shown="\"Positive\", Default" w219 {
                      tunnel: w218 -> [w224 w228]
                      tunnel: w217 -> [w223 w227]
                      tunnel: [u16 0 ("DC Param") u16 2 ("DC Param")] -> w214
                      tunnel: [u16 6 ("DC Param") u16 12 ("DC Param")] -> w213
                      frame "Positive", Default {
                        n84 = global write "_Global Configuration.vi" "Resolution 3"(w223) -> ()
                        n85 = global write "_Global Configuration.vi" "Calibration"(w224) -> ()
                      }
                      frame "Negative" {
                        n86 = global write "_Global Configuration.vi" "Calibration 3"(w228) -> ()
                        n87 = global write "_Global Configuration.vi" "Resolution 9"(w227) -> ()
                      }
                    }
                    n88 = local read "Pause"() -> (w206:bool)
                    n89 = Not(x=w206) -> (.not. x?=w205:bool)
                    n90 = And(x=w205, y=w204) -> (x .and. y?=w203:bool)
                    n91 = case shown="True" w203 {
                      frame False {
                      }
                      frame True {
                        n92 = call "_ShowMessage.vi"("Message"="Check missing peak then press Continue button." ("message")) -> ()  [unwired: 1 in, 1 out]
                      }
                    }
                    n93 = call "_Remote Communicate.vi"("DC Param"=w214, "Command"=w215) -> ("error out"=w216:errorcluster)  [unwired: 4 in, 3 out]
                    n94 = call "_Remote Communicate.vi"("error in (no error)"=w216, "DC Param"=w213, "Command"=w215) -> ()  [unwired: 3 in, 4 out]
                    n95 = Or(x=w204, y=w206) -> (x .or. y?=w208:bool)
                    n96 = Select(t=_CalibrationStep."Pause", s=w208, f=_CalibrationStep."Acquire Q1 Data") -> (s? t:f=w210:T1)
                  }
                  frame True {
                    n97 = case shown="False" w231 {
                      tunnel: [_CalibrationStep."Done" ("t") _CalibrationStep."Generate Report" ("f")] -> w232
                      tunnel: [w234 w238] -> w230
                      tunnel: w229 -> [w233 w238]
                      frame False {
                        n98 = call "_Construct Error Cluster.vi"("error in"=w233, "reason"="One or more of the calculated DAC values are out of range:\nCalibration DAC (0-262144); Resolution DAC (0-65536).", "CallingChain? (T)"=FALSE) -> ("error out"=w234:errorcluster)  [unwired: 4 in]
                      }
                      frame True {
                        # "Finish calibration"
                      }
                    }
                  }
                }
              }
              frame True {
                n99 = local read "Model Name"() -> (w254:T2)
                n100 = local read "CalOption"() -> (w253:enum32{"Positive", "Negative"})
                n101 = call "AutoDetector_GetPeak.vi"("AutoDV Info"=w246, "error in"=w256, "CalOption"=w253, "Model Name"=w254, "Current Results"=w255) -> ("error in"=w252:errorcluster, "AutoDV Info Out"=w251:T10)  [unwired: 5 in]
                n102 = call "AutoDetector_ValidatePeak.vi"("Error In"=w252, "Auto-DV Info In"=w251) -> ("Error Out"=w250:errorcluster, "Correct Run Bias Reached"=w247:bool, "Optimized DV Value"=w244:u32, "Auto-DV Info Out"=w248:T10)  [unwired: 6 in]
                n103 = local read "Pause"() -> (w241:bool)
                n104 = call "AutoDetector_RunResult.vi"("Error In"=w250, "Correct Run Bias Reached"=w247, "Optimized DV Value"=w244, "Auto-DV Info In"=w248) -> ("Error Out"=w249:errorcluster, "Next State"=w243:T1, "Auto-DV Info Out"=w245:T10)  [unwired: 5 in]
                n105 = Select(t=_CalibrationStep."Pause", s=w241, f=w243) -> (s? t:f=w242:T1)
              }
            }
            n106 = Bundle("RefMass"=w178, "MassShift"=w177) -> (→"MassShift":cluster{"RefMass":dbl[], "MassShift":dbl[]})  [unwired: 1 in]
            n107 = Bundle("RefMass"=w178, "PeakWidth"=w180) -> (→"PeakWidth":cluster{"RefMass":dbl[], "PeakWidth":dbl[]})  [unwired: 1 in]
            n108 = local read "Iteration #"() -> (w169:i32)
            n109 = Increment(x=w169) -> (x+1=w170:i32)
            n110 = local write "Iteration #"(w170) -> ()
          }
          frame "Generate Report" {
            n111 = Get Date/Time In Seconds() -> (seconds since 1Jan1904=w273:timestamp)
            n112 = property on="CalOption 2" class="Enum (strict)"() -> ("Strings []"=w266:string[])  [unwired: 2 in, 2 out]
            n113 = local read "ReportFolder"() -> (w267:path)
            n114 = Index Array(array=w266, index=w265) -> (element=w264:string)
            n115 = Format Date/Time String(time format string (%c)="%y%m%d %H%M.jpg", seconds (now)=w273) -> (date/time string=w272:string)  [unwired: 1 in]
            n116 = case shown="\"Process Q1 Data\", Default" w269 {
              tunnel: [w303 w306] -> w275
              tunnel: [_CalibrationStep."Done" ("f") _CalibrationStep."Prepare For Q2 Cal" ("f")] -> w276
              tunnel: w264 -> [w302 w308]
              frame "Process Q2 Data" {
                n117 = Concatenate Strings("Calibration Q2 " ("time format string (%c)"), w302, " Report " ("string")) -> (w303:string)
              }
              frame "Process Q1 Data", Default {
                n118 = Concatenate Strings("Calibration Q1 " ("time format string (%c)"), w308, " Report " ("string")) -> (w306:string)
              }
            }
            n119 = File/Directory Info(path=w267) -> (directory=w271:bool)  [unwired: 1 in, 6 out]
            n120 = case shown="False" w271 {
              tunnel: w267 -> [w281 w282]
              tunnel: [w280 w282] -> w270
              frame False {
                n121 = Create Folder(path (use dialog)=w281) -> (created path=w280:path)  [unwired: 2 in, 2 out]
              }
              frame True {
              }
            }
            n122 = stacked-sequence {
              tunnel: w270 -> [_ w296 _]
              tunnel: w275 -> [_ w295 _]
              tunnel: w272 -> [_ w294 _]
              tunnel: [_ w290 _] -> w268
              tunnel: w262 -> [w285 _ _]
              tunnel: [w285 _ _] -> w261
              frame #0 {
                w286 = FALSE ("Visible")
                n123 = local read "Current Results"() -> (w284:string[][])
                n124 = local write "Pages"(enum32{"Page 1", "Page 2", "Page 3", "Page 4"}."Page 1" ("Pages")) -> ()
                n125 = call "_modifyResultsStatus.vi"("Current Results In"=w284) -> ("Current Results Out"=w283:string[][])  [unwired: 10 in]
                n126 = local write "Page"(TRUE ("Page")) -> ()
                n127 = local write "Current Results"(w283) -> ()
                n128 = Wait (ms)(milliseconds to wait=u32 280) -> ()  [unwired: 1 out]
                n129 = property on="Calibration State" class="Enum (strict)"("Visible"=w286) -> ()  [unwired: 2 in, 2 out]
                n130 = property on="Current Scan #" class="DigNum (strict)"("Visible"=w286) -> ()  [unwired: 2 in, 2 out]
                n131 = property on="Pause" class="Bool (strict)"("Visible"=w286) -> ()  [unwired: 2 in, 2 out]
                n132 = property on="Print" class="Bool"("Visible"=w286) -> ()  [unwired: 2 in, 2 out]
                n133 = property on="Iteration #" class="DigNum (strict)"("Visible"=w286) -> ()  [unwired: 2 in, 2 out]
                n134 = property on="GotoPg1" class="Bool"("Visible"=w286) -> ()  [unwired: 2 in, 2 out]
                n135 = property on="GotoPg2" class="Bool"("Visible"=w286) -> ()  [unwired: 2 in, 2 out]
              }
              frame #1 {
                n136 = Concatenate Strings(w295, w294) -> (w297:string)
                n137 = invoke class="VI" method="FP.Get Image"("visible area only"=FALSE ("Visible Area Only")) -> ("image data"=w299:T17)  [unwired: 5 in, 5 out]
                n138 = Build Path(base path=w296, name or relative path=w297) -> (appended path=w290:path)
                n139 = call <vilib>:"Write JPEG File.vi"("image data"=w299, "path to JPEG file"=w290) -> ("error out"=w291:errorcluster)  [unwired: 1 in, 8 out]
                n140 = Path To String(path=w290) -> (string=w293:string)
                n141 = call "_Log Events.vi"("error in (no error)"=w291, "Event"=w293, "Log Command"=_Log_Command."Write") -> ()  [unwired: 5 in, 2 out]
              }
              frame #2 {
                w300 = TRUE ("Visible")
                n142 = property on="Calibration State" class="Enum (strict)"("Visible"=w300) -> ()  [unwired: 2 in, 2 out]
                n143 = property on="Pause" class="Bool (strict)"("Visible"=w300) -> ()  [unwired: 2 in, 2 out]
                n144 = property on="Print" class="Bool"("Visible"=w300) -> ()  [unwired: 2 in, 2 out]
                n145 = property on="Current Scan #" class="DigNum (strict)"("Visible"=w300) -> ()  [unwired: 2 in, 2 out]
                n146 = property on="Iteration #" class="DigNum (strict)"("Visible"=w300) -> ()  [unwired: 2 in, 2 out]
              }
            }
            n147 = case shown="\"Process Q1 Data\", Default" w269 {
              tunnel: w268 -> [w278 w279]
              frame "Process Q1 Data", Default {
                "Q1ReportPage" <- w278
              }
              frame "Process Q2 Data" {
                "Q2ReportPage" <- w279
              }
            }
          }
          frame "Prepare For Q2 Cal" {
            # "Save Q1 calibration result table\nLoad the previous Q2 calibration result table"
            n148 = case shown="\"Positive\", Default" w332 {
              tunnel: ["For Q2 Positive Mode" ("ScanMode") "For Q2 Negative Mode" ("ScanMode")] -> w323
              tunnel: ["Q2, Positive" ("time format string (%c)") "Q2, Negative" ("time format string (%c)")] -> w317
              tunnel: ["Q2 PPG POS Default.method" ("time format string (%c)") "Q2 PPG NEG Default.method" ("time format string (%c)")] -> w319
              tunnel: ["PositiveQ2Result" ("section") "NegativeQ2Result" ("section")] -> w311
              frame "Positive", Default {
              }
              frame "Negative" {
              }
            }
            n149 = local read "Current Results"() -> (w312:string[][])
            "Q1 Data" <- w312
            n150 = call "_Open Preference File.vi"() -> ("error"=w330:errorcluster, "refnum"=w331:T16)  [unwired: 3 in, 3 out]
            n151 = local read "SystemInfo"() -> (w320:string)
            n152 = local write "ScanMode"(w323) -> ()
            n153 = call "_ReplaceInfoString.vi"("Value"=w319, "Key"="Method", "SystemInfo"=w320) -> ("SystemInfoOut"=w318:string)  [unwired: 4 in]
            n154 = call-poly <vilib>:"Read Key.vi"("section"="AutoCal", "error in (no error)"=w330, "default value"="", "key"=w311, "refnum"=w331) -> ("error out"=w328:errorcluster, "value"=w325:string, "refnum out"=w329:T16)  [unwired: 3 in, 1 out]
            n155 = call "_ReplaceInfoString.vi"("Value"=w317, "Key"="Scan Mode", "SystemInfo"=w318) -> ("SystemInfoOut"=w315:string)  [unwired: 4 in]
            n156 = Unflatten From String(type=w312, binary string=w325) -> (value=w324:string[][])  [unwired: 3 in, 2 out]
            n157 = local write "Previous Auto Calibration Results"(w324) -> ()
            n158 = call <vilib>:"Close Config Data.vi"("error in (no error)"=w328, "refnum"=w329) -> ()  [unwired: 1 in, 9 out]
            n159 = local write "SystemInfo"(w315) -> ()
          }
          frame "Read Q2 Method" {
            # "Load Q2 method from a file\nValidate the method for AutoCal\nConvert method to Sniffer format\nDisplay the lens values\nPrepare for data acquisition"
            n160 = local read "Q2 Method"() -> (w343:path)
            n161 = local read "MassReference"() -> (w346:cluster{"Mass":dbl, "Use":bool}[])
            n162 = call "_ReadCalMethod.vi"("HasESI2"=w351, "HasESI1"=w352, "Method Path"=w343) -> ("error out"=w350:errorcluster, "UseESI1"=w353:bool, "GUI Method"=w349:T3)  [unwired: 2 in]
            n163 = call "_ValidateRefPeaks.vi"("error in (no error)"=w350, "MassReference"=w346, "Method"=w349) -> ("error out"=w348:errorcluster)  [unwired: 4 in]
            n164 = case shown="No Error" w348 {
              selector: w348 -> [w355 w374]
              tunnel: [_CalibrationStep."Acquire Q2 Data" ("f") _CalibrationStep."Done" ("f")] -> w354
              tunnel: w349 -> [w366 _]
              tunnel: w353 -> [w367 _]
              tunnel: w347 -> [_ w375]
              tunnel: w346 -> [w358 _]
              tunnel: [w356 w375] -> w345
              tunnel: [w355 w374] -> w342
              frame No Error {
                n165 = local write "Method"(w366) -> ()
                n166 = local write "UsingESI1"(w367) -> ()
                n167 = call "_GetParameterList.vi"("GUI Method"=w366) -> ("Detector"=w363:string[][], "Source"=w364:string[][], "Instrument"=w365:string[][], "Resolution"=w360:string[][])  [unwired: 3 in, 1 out]
                n168 = Array Size(array=w358) -> (size(s)=w359:i32)
                n169 = local read "SystemInfo"() -> (w362:string)
                n170 = local write "Instrument"(w365) -> ()
                n171 = local write "Source"(w364) -> ()
                n172 = local write "Detector"(w363) -> ()
                n173 = Initialize Array(T11 {"RefMass"=0.0, "MassFound"=0.0, "MassShift"=0.0, "PeakWidth"=0.0, "CalDAC"=0.0, "CalSlope"=0.0, "ResDAC"=0.0, "ResSlope"=0.0, "Status"=enum."Found", "CalOK"=FALSE, "ResOK"=FALSE, "PeakHeight"=0.0} ("CalResult"), w359) -> (w356:T11[])
                n174 = local write "Resolution"(w360) -> ()
                n175 = local write "Iteration #"(0 ("Iteration #")) -> ()
                n176 = Select(t="ESI 1", s=w367, f="ESI 2") -> (s? t:f=w368:string)
                n177 = call "_ReplaceInfoString.vi"("Value"=w368, "Key"="Source", "SystemInfo"=w362) -> ("SystemInfoOut"=w372:string)  [unwired: 4 in]
                n178 = local write "SystemInfo"(w372) -> ()
              }
              frame Error {
              }
            }
          }
          frame "Acquire Q2 Data" {
            n179 = local read "Method"() -> (w385:T3)
            n180 = control-ref of="Pause"() -> (w382:refnum<vi>)
            n181 = call "_RunCalMethod.vi"("Method"=w385, "millisecond timer value"=w377, "Pause"=w382) -> ("error out"=w384:errorcluster)  [unwired: 4 in]
            n182 = Select(t=_CalibrationStep."Done", s=w384, f=_CalibrationStep."Process Q2 Data") -> (s? t:f=w383:T1)
          }
          frame "Process Q2 Data" {
            n183 = local read "MassReference"() -> (w412:cluster{"Mass":dbl, "Use":bool}[])
            n184 = case shown="\"Negative\"" w411 {
              tunnel: [w452 w454] -> w410
              tunnel: [w451 w453] -> w409
              frame "Positive", Default {
                n185 = global read "_Global Configuration.vi" "Calibration 2"() -> (w452:dbl[][])
                n186 = global read "_Global Configuration.vi" "Resolution 4"() -> (w451:dbl[][])
              }
              frame "Negative" {
                n187 = global read "_Global Configuration.vi" "Resolution 10"() -> (w453:dbl[][])
                n188 = global read "_Global Configuration.vi" "Calibration 4"() -> (w454:dbl[][])
              }
            }
            n189 = local read "PeakSearchParameters"() -> (w413:dbl[])
            n190 = call "_ProcessCalData.vi"("CalResultIn"=w391, "Resolution"=w409, "Calibration"=w410, "MassReference"=w412, "PeakSearchParameters"=w413) -> ("ResolutionOut"=w407:dbl[][], "CalibrationOut"=w408:dbl[][], "ResOK"=w405:bool, "CalOK"=w406:bool, "AllFound"=w398:bool, "CalResultOut"=w390:T11[], "AllValid"=w396:bool)
            n191 = And(x=w406, y=w405) -> (x .and. y?=w388:bool)
            n192 = global read "_Global Configuration.vi" "Sim"() -> (w386:bool)
            n193 = call "_GenerateResultTable.vi"("CalResults"=w390) -> ("ResultTable"=w404:string[][], "RefMass"=w401:dbl[], "MassShift"=w402:dbl[], "PeakWidth"=w403:dbl[])
            n194 = local write "Current Results"(w404) -> ()
            n195 = Or(x=w388, y=w386) -> (x .or. y?=w387:bool)
            n196 = case shown="True" w387 {
              tunnel: w411 -> [w430 _]
              tunnel: w408 -> [w429 _]
              tunnel: w407 -> [w428 _]
              tunnel: [w421 w443] -> w397
              tunnel: w398 -> [w419 _]
              tunnel: w396 -> [_ w442]
              tunnel: [w418 w441] -> w395
              tunnel: w394 -> [w418 w440]
              frame False {
                w426 = _RT_Command."Update Table" ("Command")
                # "Update the modified calibration and resolution tables\nRepeat the calibration cycle."
                n197 = Not(x=w419) -> (.not. x?=w415:bool)
                n198 = local read "Pause"() -> (w416:bool)
                n199 = case shown="\"Negative\"" w430 {
                  tunnel: w429 -> [w435 w439]
                  tunnel: w428 -> [w434 w438]
                  tunnel: [u16 1 ("DC Param") u16 3 ("DC Param")] -> w425
                  tunnel: [u16 7 ("DC Param") u16 13 ("DC Param")] -> w424
                  frame "Positive", Default {
                    n200 = global write "_Global Configuration.vi" "Calibration 2"(w435) -> ()
                    n201 = global write "_Global Configuration.vi" "Resolution 4"(w434) -> ()
                  }
                  frame "Negative" {
                    n202 = global write "_Global Configuration.vi" "Resolution 10"(w438) -> ()
                    n203 = global write "_Global Configuration.vi" "Calibration 4"(w439) -> ()
                  }
                }
                n204 = Not(x=w416) -> (.not. x?=w417:bool)
                n205 = And(x=w417, y=w415) -> (x .and. y?=w414:bool)
                n206 = case shown="True" w414 {
                  frame False {
                  }
                  frame True {
                    n207 = call "_ShowMessage.vi"("Message"="Check missing peak then press Continue button." ("message")) -> ()  [unwired: 1 in, 1 out]
                  }
                }
                n208 = call "_Remote Communicate.vi"("DC Param"=w425, "Command"=w426) -> ("error out"=w427:errorcluster)  [unwired: 4 in, 3 out]
                n209 = call "_Remote Communicate.vi"("error in (no error)"=w427, "DC Param"=w424, "Command"=w426) -> ()  [unwired: 3 in, 4 out]
                n210 = Or(x=w415, y=w416) -> (x .or. y?=w420:bool)
                n211 = Select(t=_CalibrationStep."Pause", s=w420, f=_CalibrationStep."Acquire Q2 Data") -> (s? t:f=w421:T1)
              }
              frame True {
                n212 = case shown="False" w442 {
                  tunnel: [_CalibrationStep."Done" ("t") _CalibrationStep."Generate Report" ("f")] -> w443
                  tunnel: [w445 w449] -> w441
                  tunnel: w440 -> [w444 w449]
                  frame False {
                    n213 = call "_Construct Error Cluster.vi"("error in"=w444, "reason"="One or more of the calculated DAC values are out of range:\nCalibration DAC (0-262144); Resolution DAC (0-65536).", "CallingChain? (T)"=FALSE) -> ("error out"=w445:errorcluster)  [unwired: 4 in]
                  }
                  frame True {
                    # "Finish calibration"
                  }
                }
              }
            }
            n214 = Bundle("RefMass"=w401, "MassShift"=w402) -> (w399:cluster{"RefMass":dbl[], "MassShift":dbl[]})  [unwired: 1 in]
            n215 = Bundle("RefMass"=w401, "PeakWidth"=w403) -> (w400:cluster{"RefMass":dbl[], "PeakWidth":dbl[]})  [unwired: 1 in]
            n216 = local write "MassShift"(w399) -> ()
            n217 = local write "PeakWidth"(w400) -> ()
            n218 = local read "Iteration #"() -> (w392:i32)
            n219 = Increment(x=w392) -> (x+1=w393:i32)
            n220 = local write "Iteration #"(w393) -> ()
          }
          frame "Done" {
            # "Wait until the user exits the window."
            n221 = case shown="No Error" w462 {
              selector: w462 -> [_ w518]
              tunnel: w465 -> [w476 _]
              tunnel: [w472 w519] -> w463
              tunnel: w461 -> [w475 _]
              tunnel: w460 -> [w468 _]
              tunnel: w458 -> [w473 _]
              tunnel: w457 -> [w474 _]
              tunnel: w455 -> [w466 _]
              frame No Error {
                n222 = Not Equal?(x=_CalibrationStep."Export Optimization" ("Next State"), y=w468) -> (x != y?=w467:bool)
                n223 = Not Equal?(x=w475, y=w468) -> (x != y?=w470:bool)
                n224 = And(x=w467, y=w470) -> (x .and. y?=w471:bool)
                n225 = case shown="True" w471 {
                  tunnel: w476 -> [_ w486]
                  tunnel: w474 -> [_ w485]
                  tunnel: w473 -> [_ w483]
                  tunnel: [w477 _] -> w472
                  tunnel: w466 -> [_ w481]
                  frame False {
                    n226 = while {
                      tunnel: [w478] -> w477
                      stop <- w478 stop-if-true
                      # "Wait until the user press close button or exits the window."
                      n227 = call "_Remote Communicate.vi"("Command"=_RT_Command."Get Status") -> ()  [unwired: 5 in, 4 out]
                      n228 = local read "Quit"() -> (w478:bool)
                      n229 = Wait (ms)(milliseconds to wait=u32 380) -> ()  [unwired: 1 out]
                    }
                  }
                  frame True {
                    n230 = call "ReviewReports.vi"("Q2Report"=w483, "Q1Report"=w485) -> ("Accepted"=w484:bool)  [unwired: 5 in]
                    n231 = case shown="True" w484 {
                      tunnel: w486 -> [_ w488]
                      tunnel: w481 -> [_ w487]
                      frame False {
                      }
                      frame True {
                        n232 = case shown="\"Negative\"" w488 {
                          tunnel: ["PositiveQ2Result" ("section") "NegativeQ2Result" ("section")] -> w510
                          frame "Positive", Default {
                          }
                          frame "Negative" {
                          }
                        }
                        n233 = local read "Current Results"() -> (w507:string[][])
                        n234 = local read "ParmeterFolder"() -> (w490:path)
                        n235 = call "_Open Preference File.vi"() -> ("error"=w504:errorcluster, "refnum"=w505:T16)  [unwired: 3 in, 3 out]
                        n236 = File/Directory Info(path=w490) -> (directory=w503:bool)  [unwired: 1 in, 6 out]
                        n237 = Get Date/Time In Seconds() -> (seconds since 1Jan1904=w495:timestamp)
                        n238 = Flatten To String(anything=w507) -> (data string=w506:string)  [unwired: 3 in, 2 out]
                        n239 = call-poly <vilib>:"Write Key.vi"("section"="AutoCal", "error in (no error)"=w504, "value"=w506, "key"=w510, "refnum"=w505) -> ("error out"=w508:errorcluster, "refnum out"=w509:T16)  [unwired: 4 in, 1 out]
                        n240 = case shown="False" w503 {
                          tunnel: w490 -> [w513 w514]
                          tunnel: [w512 w514] -> w498
                          frame False {
                            n241 = Create Folder(path (use dialog)=w513) -> (created path=w512:path)  [unwired: 2 in, 2 out]
                          }
                          frame True {
                          }
                        }
                        n242 = Format Date/Time String(time format string (%c)="My Tables-%y%m%d-%H%M.tbl", seconds (now)=w495) -> (date/time string=w500:string)  [unwired: 1 in]
                        n243 = call <vilib>:"Close Config Data.vi"("error in (no error)"=w508, "refnum"=w509) -> ()  [unwired: 1 in, 9 out]
                        n244 = Build Path(base path=w498, name or relative path=w500) -> (appended path=w496:path)
                        n245 = local read "Q1 Data"() -> (w489:string[][])
                        n246 = Format Into String(initial string="AutoCal completed successfully, the latest table has been saved to, %s.", w496) -> (resulting string=w493:string)  [unwired: 2 in, 1 out]
                        n247 = Path To String(path=w496) -> (string=w499:string)
                        n248 = call "_Save All Tables.vi"("FilePath(My Table.tbl)"=w499, "SaveOption (Temporary File)"=_SaveOption."Full Path" ("Use temporary file (F)")) -> ("error out"=w492:errorcluster)  [unwired: 1 in, 4 out]
                        n249 = call "Write Q1 Data.vi"("Q1 Data in"=w489, "section"=w487, "CalOption"=w488) -> ()  [unwired: 9 in]
                        n250 = call "_Log Events.vi"("error in (no error)"=w492, "Event"=w493, "Log Command"=_Log_Command."Write") -> ()  [unwired: 5 in, 2 out]
                        n251 = property class="VI"("Front Panel Window:Title"="Auto Calibration Completed") -> ()  [unwired: 2 in, 2 out]
                      }
                    }
                    "Completed" <- TRUE ("Accepted")
                  }
                }
              }
              frame Error {
                w519 = TRUE
                n252 = Unbundle By Name(w518) -> ("source"=w517:string)
                n253 = call "_ShowMessage.vi"("Message"=w517) -> ()  [unwired: 1 in, 1 out]
                n254 = property class="VI"("Front Panel Window:Title"="Auto Calibration Aborting Due to Error") -> ()  [unwired: 2 in, 2 out]
                n255 = local write "Quit"(w519) -> ()
              }
            }
            n256 = property on="Pause" class="Bool (strict)"("Visible"=FALSE) -> ()  [unwired: 2 in, 2 out]
          }
          frame "Pause" {
            n257 = case shown="\"Process Q1 Data\", Default" w525 {
              tunnel: [_CalibrationStep."Acquire Q2 Data" ("f") _CalibrationStep."Acquire Q1 Data" ("f")] -> w524
              frame "Process Q2 Data" {
              }
              frame "Process Q1 Data", Default {
              }
            }
            n258 = stacked-sequence {
              tunnel: [_ w528 _] -> w523
              frame #0 {
                n259 = property on="Pause" class="Bool (strict)"("Value"=TRUE ("Pause")) -> ()  [unwired: 2 in, 2 out]
              }
              frame #1 {
                n260 = while {
                  tunnel: [w529] -> w528
                  stop <- w532 stop-if-true
                  # "Wait until the user press Continue button or exits the window."
                  n261 = call "_Remote Communicate.vi"("Command"=_RT_Command."Get Status") -> ()  [unwired: 5 in, 4 out]
                  n262 = local read "Quit"() -> (w529:bool)
                  n263 = Not(x="Pause") -> (.not. x?=w533:bool)
                  n264 = Or(x=w533, y=w529) -> (x .or. y?=w532:bool)
                  n265 = Wait (ms)(milliseconds to wait=u32 380) -> ()  [unwired: 1 out]
                }
              }
              frame #2 {
                n266 = property on="Pause" class="Bool (strict)"("Value"=FALSE ("Pause")) -> ()  [unwired: 2 in, 2 out]
              }
            }
          }
          frame "Export Optimization" {
            n267 = Unbundle By Name(w554) -> ("Optimization Run Bias"=w539:u32, "Run Bias Info"=w553:T9[])
            n268 = Format Into String(format string="Optimization Run Bias of %d  found. Accept new Value?", w539) -> (resulting string=w546:string)  [unwired: 2 in, 1 out]
            n269 = call <vilib>:"Three Button Dialog.vi"("Allow user to close window? (TRUE)"=FALSE, "Window Title (\"\")"="AutoDV Complete" ("Window Title (\"\")"), "Right Button Text (\"Cancel\")"="No" ("Right Button Text (\"Cancel\")"), "Center Button Text (\"No\")"="Yes and Run AutoCal" ("Center Button Text (\"No\")"), "Left Button Text (\"Yes\")"="Yes and Exit" ("Left Button Text (\"Yes\")"), "message"=w546) -> ("Which Button?"=w540:T18)  [unwired: 5 in]
            n270 = case shown="\"Left Button\", \"Center Button\"" w540 {
              selector: w540 -> [_ w558]
              tunnel: w553 -> [_ w560]
              tunnel: [_CalibrationStep."Done" ("f") w564] -> w550
              tunnel: w539 -> [_ w561]
              tunnel: w549 -> [w556 w562]
              tunnel: [w556 w559] -> w548
              tunnel: [_ w563] -> w538
              frame "Right Button", Default {
              }
              frame "Left Button", "Center Button" {
                n271 = call "_Accept AutoDV results.vi"("error in (no error)"=w562, "Run Bias Info"=w560, "Optimization Run Bias"=w561) -> ("error out"=w559:errorcluster)  [unwired: 8 in]
                n272 = case shown="\"Center Button\"" w558 {
                  tunnel: [_CalibrationStep."Get Cal Files" ("f") _CalibrationStep."Export Optimization" ("f")] -> w564
                  tunnel: [_ w566] -> w563
                  frame "Center Button" {
                  }
                  frame "Left Button", Default {
                    w566 = TRUE ("Allow user to close window? (TRUE)")
                    n273 = local write "Quit"(w566) -> ()
                  }
                }
              }
            }
            n274 = Bundle By Name(cluster=w554, "Run Optimization Proc"=FALSE) -> (w552:T10)
          }
        }
        n275 = local read "Quit"() -> (w80:bool)
        n276 = Or(x=w81, y=w80) -> (x .or. y?=w79:bool)
        "Calibration State" <- w82
      }
      "error out" <- w56
      n277 = while {
        shift-right: [w568] -> _
        shift-left: w53 -> [w569]
        stop <- w570 stop-if-true
        n278 = event shown="[5] \"Print\": Value Change" {
          selector: _ -> [_ _ _ _ _ _ _]
          dyn-events: _ -> [_ _ _ _ _ _ _]
          timeout: 180 -> [_ _ _ _ _ _ _]
          tunnel: [w573 w601 _ _ _ _ _] -> w570
          tunnel: w569 -> [w572 w593 w634 w641 w647 w660 w661]
          tunnel: [w572 w592 w634 w641 w647 w660 w661] -> w568
          event Panel Close? {
            n279 = event-data() -> ()  [unwired: 2 out]
            n280 = local read "Calibration State"() -> (w576:T1)
            n281 = Equal?(x=w576, y=_CalibrationStep."Done") -> (x = y?=w574:bool)
            n282 = case shown="False" w574 {
              selector: w574 -> [_ w591]
              tunnel: [w583 w591] -> w573
              frame False {
                n283 = local read "Run Optimization Proc"() -> (w578:bool)
                n284 = Select(t="Auto DV" ("source"), s=w578, f="Auto calibration" ("source")) -> (s? t:f=w581:string)
                n285 = Concatenate Strings(w581, " is in progress, are you sure you want to abort?" ("message")) -> (w582:string)
                n286 = Two Button Dialog(message=w582, 1:"No" ("F button name (\"Cancel\")"), 2:"Yes" ("T button name (\"OK\")")) -> (T button?=w583:bool)
                n287 = case shown="True" w583 {
                  selector: w583 -> [_ w587]
                  frame False {
                  }
                  frame True {
                    n288 = local write "Quit"(w587) -> ()
                    n289 = global write "_Global Configuration.vi" "Run"(FALSE ("Run")) -> ()
                    n290 = call "_Log Events.vi"("Event"="AutoCal was aborted by user.", "Log Command"=_Log_Command."Write") -> ()  [unwired: 6 in, 2 out]
                  }
                }
              }
              frame True {
                n291 = local write "Quit"(w591) -> ()
              }
            }
            n292 = event-data("Discard?"=TRUE) -> ()  [unwired: 1 in, 1 out]
          }
          event Timeout {
            n293 = event-data() -> ()  [unwired: 2 out]
            n294 = local read "Current Scan #"() -> (w598:i32)
            n295 = local read "MassReference"() -> (w595:cluster{"Mass":dbl, "Use":bool}[])
            n296 = call "_Current Data Global.vi"("Operation"=_Data_Operation."Get Data") -> ("CurrentData"=w600:T19[])  [unwired: 3 in, 3 out]
            n297 = Index Array(array=w600) -> (element=w596:T19)  [unwired: 1 in]
            n298 = Unbundle By Name(w596) -> ("Scan#"=w594:i32)
            n299 = Equal?(x=w594, y=w598) -> (x = y?=w597:bool)
            n300 = case shown="True" w597 {
              tunnel: w596 -> [w621 _]
              tunnel: w595 -> [w604 _]
              tunnel: w594 -> [w603 _]
              tunnel: w593 -> [w602 w625]
              tunnel: [w602 w626] -> w592
              frame False {
                n301 = local write "Current Scan #"(w603) -> ()
                n302 = control-ref of="MR 5"() -> (w611:refnum<vi>)
                n303 = control-ref of="MR 1"() -> (w612:refnum<vi>)
                n304 = call "_UpdateSpectralPlot.vi"("MassRange# (0)"=4, "MassReference"=w604, "Current Data"=w621, "Display Refnum"=w611) -> ()  [unwired: 5 in]
                n305 = call "_UpdateSpectralPlot.vi"("MassRange# (0)"=0, "MassReference"=w604, "Current Data"=w621, "Display Refnum"=w612) -> ()  [unwired: 5 in]
                n306 = control-ref of="MR 2"() -> (w610:refnum<vi>)
                n307 = control-ref of="MR 6"() -> (w609:refnum<vi>)
                n308 = call "_UpdateSpectralPlot.vi"("MassRange# (0)"=1, "MassReference"=w604, "Current Data"=w621, "Display Refnum"=w610) -> ()  [unwired: 5 in]
                n309 = call "_UpdateSpectralPlot.vi"("MassRange# (0)"=5, "MassReference"=w604, "Current Data"=w621, "Display Refnum"=w609) -> ()  [unwired: 5 in]
                n310 = control-ref of="MR 3"() -> (w608:refnum<vi>)
                n311 = control-ref of="MR 7"() -> (w606:refnum<vi>)
                n312 = call "_UpdateSpectralPlot.vi"("MassRange# (0)"=6, "MassReference"=w604, "Current Data"=w621, "Display Refnum"=w606) -> ()  [unwired: 5 in]
                n313 = call "_UpdateSpectralPlot.vi"("MassRange# (0)"=2, "MassReference"=w604, "Current Data"=w621, "Display Refnum"=w608) -> ()  [unwired: 5 in]
                n314 = control-ref of="MR 8"() -> (w605:refnum<vi>)
                n315 = control-ref of="MR 4"() -> (w607:refnum<vi>)
                n316 = call "_UpdateSpectralPlot.vi"("MassRange# (0)"=3, "MassReference"=w604, "Current Data"=w621, "Display Refnum"=w607) -> ()  [unwired: 5 in]
                n317 = call "_UpdateSpectralPlot.vi"("MassRange# (0)"=7, "MassReference"=w604, "Current Data"=w621, "Display Refnum"=w605) -> ()  [unwired: 5 in]
              }
              frame True {
                n318 = Tick Count (ms)() -> (millisecond timer value=w627:u32)
                n319 = Subtract(x=w627, y=w625) -> (x-y=w630:u32)
                n320 = global read "_Global Configuration.vi" "Run"() -> (w623:bool)
                n321 = Not(x=w623) -> (.not. x?=w622:bool)
                n322 = Greater?(x=w630, y=u32 3000) -> (0:w628:bool)
                n323 = And(x=w622, y=w628) -> (x .and. y?=w624:bool)
                n324 = case shown="True" w624 {
                  tunnel: [w631 w632] -> w626
                  tunnel: w625 -> [w631 _]
                  frame False {
                  }
                  frame True {
                    n325 = call "_Remote Communicate.vi"("Command"=_RT_Command."Get Status") -> ()  [unwired: 5 in, 4 out]
                    n326 = Tick Count (ms)() -> (millisecond timer value=w632:u32)
                  }
                }
              }
            }
            n327 = local read "Quit"() -> (w601:bool)
          }
          event "Init": Value Change {
            w637 = dbl[] []
            n328 = event-data() -> ()  [unwired: 4 out]
            n329 = Bundle(w637, w637) -> (→"MR 1" →"MR 2" →"MR 3" →"MR 4" →"MR 5" →"MR 6" →"MR 7" →"MR 8":cluster{dbl[], dbl[]})  [unwired: 1 out]
            n330 = call "_Log Events.vi"("Event"="An auto calibration run has been started.", "Log Command"=_Log_Command."Write") -> ()  [unwired: 6 in, 2 out]
            "Init" <- FALSE ("Init")
            "Current Scan #" <- 0 ("Scan#")
          }
          event "Page": Value Change {
            n331 = event-data() -> ("NewVal"=w642:bool)  [unwired: 1 out]
            n332 = local write "Page"(w642) -> ()
            n333 = Select(t=enum32{"Page 1", "Page 2", "Page 3", "Page 4"}."Page 1" ("Pages"), s=w642, f=enum32{"Page 1", "Page 2", "Page 3", "Page 4"}."Page 2" ("Pages")) -> (s? t:f=w644:enum32{"Page 1", "Page 2", "Page 3", "Page 4"})
            n334 = local write "Pages"(w644) -> ()
            n335 = Not(x=w642) -> (.not. x?=w643:bool)
            n336 = property on="GotoPg1" class="Bool"("Visible"=w643) -> ()  [unwired: 2 in, 2 out]
            n337 = property on="GotoPg2" class="Bool"("Visible"=w642) -> ()  [unwired: 2 in, 2 out]
          }
          event "GotoPg2", "GotoPg1": Value Change {
            n338 = event-data() -> ()  [unwired: 2 out]
            n339 = case shown="True" "GotoPg2" {
              frame False {
              }
              frame True {
                n340 = property on="Page" class="Bool (strict)"("Val(Sgnl)"=FALSE ("Value (Signaling)")) -> ()  [unwired: 2 in, 2 out]
              }
            }
            n341 = case shown="True" "GotoPg1" {
              frame False {
              }
              frame True {
                n342 = property on="Page" class="Bool (strict)"("Val(Sgnl)"=TRUE ("Value (Signaling)")) -> ()  [unwired: 2 in, 2 out]
              }
            }
          }
          event "Print": Value Change {
            # "Had to call this VI asynchroniusly otherwise it would pause the graphs being updated"
            n343 = event-data() -> ()  [unwired: 2 out]
            n344 = vi-ref "Print AutoCal FP.vi"() -> (w656:refnum<vi>)
            n345 = property class="VI Interface Type 0"(reference=w656) -> (error out=w659:errorcluster, "Path"=w653:path)  [unwired: 1 in, 1 out]
            n346 = Open VI Reference(type specifier VI Refnum (for type only)=w656, vi path=w653, options=128, error in (no error)=w659) -> (vi reference=w657:refnum<vi>, error out=w658:errorcluster)  [unwired: 2 in]
            n347 = control-ref of="This VI"() -> (w654:refnum<vi>)
            n348 = call-by-ref "Start Asynchronous Call"(reference=w657, error in=w658, "name or relative path"="AutoCal.jpg", "VI in"=w654) -> ()  [unwired: 10 in, 2 out]
          }
          event "Pause": Value Change {
            n349 = event-data() -> ("NewVal"=w664:bool)  [unwired: 1 out]
            n350 = global read "_Global Configuration.vi" "Run"() -> (w663:bool)
            n351 = And(x=w664, y=w663) -> (x .and. y?=w662:bool)
            n352 = case shown="True" w662 {
              frame False {
              }
              frame True {
                # "abort the current run cycle when user press pause button"
                n353 = global write "_Global Configuration.vi" "Run"(FALSE ("Run")) -> ()
              }
            }
          }
        }
      }
      "CalOption 2" <- w64
    }
    frame #2 {
      n354 = local read "Quit"() -> (w666:bool)
      n355 = local read "error out"() -> (w670:errorcluster)
      n356 = Unbundle By Name(w670) -> ("status"=w669:bool)
      n357 = Or(x=w669, y=w666) -> (x .or. y?=w668:bool)
      n358 = case shown="True" w668 {
        tunnel: w667 -> [_ w671]
        frame False {
        }
        frame True {
          w675 = TRUE ("Check Exist (F)")
          n359 = local read "oldTablePath"() -> (w673:path)
          n360 = call "_Validate Path.vi"("Check Type (F)"=w675, "Check Exist (F)"=w675, "Type (isd)"="tbl", "path"=w673) -> ("Valid"=w672:bool)
          n361 = case shown="True" w672 {
            tunnel: w671 -> [_ w677]
            frame False {
            }
            frame True {
              # "Review Reports takes care of reverting changes"
              n362 = local read "Calibration State"() -> (w676:T1)
              n363 = case shown="Default" w676 {
                tunnel: w677 -> [w682 _]
                frame Default {
                  n364 = call "_ShowMessage.vi"("TwoButton? (F)"=TRUE, "Message"="Do you want to keep the current calibration results after aborting?" ("message")) -> ("Ok?"=w678:bool)
                  n365 = disable-structure shown="Enabled" {
                    disable-tunnel: [w684 w689] -> w681
                    disable-tunnel: w678 -> [w683 w689]
                    frame Disabled {
                      n366 = case shown="True" w683 {
                        selector: w683 -> [_ w686]
                        tunnel: [_ w688] -> w684
                        frame False {
                        }
                        frame True {
                          n367 = call "Read AutoCal Password.vi"() -> ("Password"=w685:string)  [unwired: 10 in, 1 out]
                          n368 = call "AutoCal Password.vi"("IonSniffer777"=w685) -> ("Valid"=w687:bool)  [unwired: 5 in, 1 out]
                          n369 = And(x=w687, y=w686) -> (x .and. y?=w688:bool)
                        }
                      }
                    }
                    frame Enabled {
                    }
                  }
                  n370 = case shown="False" w681 {
                    tunnel: w682 -> [_ _]
                    frame False {
                      # "Revert the changes in case of an error"
                      n371 = call "_Load All Tables.vi"("Use temporary file (F)"=TRUE) -> ()  [unwired: 7 out]
                    }
                    frame True {
                    }
                  }
                }
                frame "Done" {
                }
              }
            }
          }
        }
      }
    }
  }
